vi "CSV_Image_Data_Create.vi"() -> ()   [LabVIEW 2022 SP3]
uses:
  <vilib>/Utility/file.llb/Write Delimited Spreadsheet (string).vi
panel:
  out "error out":errorcluster
  in  "error in (no error)":errorcluster
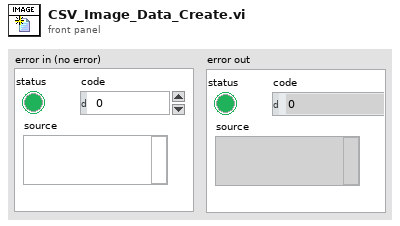
[diagram p1: front panel]
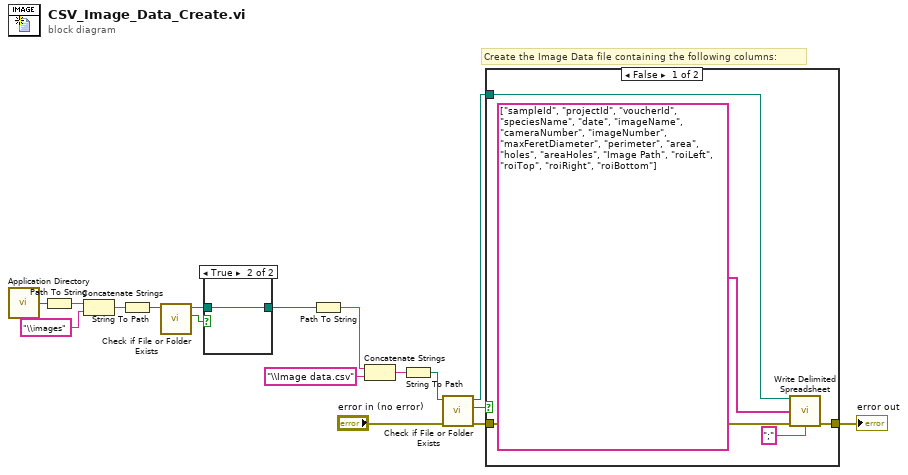
[diagram p0: block diagram]
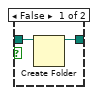
[diagram p2: hidden frame]
diagram:
  # "Create the Image Data file containing the following columns:"
  n1 = call <vilib>:"Application Directory.vi"() -> ("Application Directory"=w8:path)
  n2 = Path To String(path=w8) -> (string=w7:string)
  n3 = Concatenate Strings(w7, "\\images") -> (w5:string)
  n4 = String To Path(string=w5) -> (path=w4:path)
  n5 = call <vilib>:"Check if File or Folder Exists.vi"("path"=w4) -> ("file or folder exists?"=w3:bool, "dup path"=w2:path)  [unwired: 8 in, 1 out]
  n6 = case shown="True" w3 {
    tunnel: w2 -> [w19 w20]
    tunnel: [w18 w20] -> w1
    frame False {
      n7 = Create Folder(path (use dialog)=w19) -> (created path=w18:path)  [unwired: 2 in, 2 out]
    }
    frame True {
    }
  }
  n8 = Path To String(path=w1) -> (string=w17:string)
  n9 = Concatenate Strings(w17, "\\Image data.csv") -> (w15:string)
  n10 = String To Path(string=w15) -> (path=w14:path)
  n11 = call <vilib>:"Check if File or Folder Exists.vi"("error in (no error)"="error in (no error)", "path"=w14) -> ("error out"=w11:errorcluster, "file or folder exists?"=w13:bool, "dup path"=w12:path)  [unwired: 7 in]
  n12 = case shown="False" w13 {
    tunnel: w12 -> [w24 _]
    tunnel: w11 -> [w23 w26]
    tunnel: [w22 w26] -> w9
    frame False {
      n13 = call-poly <vilib>:"Write Delimited Spreadsheet.vi"("file path (dialog if empty)"=w24, "1D data"=string[] ["sampleId", "projectId", "voucherId", "speciesName", "date", "imageName", "cameraNumber", "imageNumber", "maxFeretDiameter", "perimeter", "area", "holes", "areaHoles", "Image Path", "roiLeft", "roiTop", "roiRight", "roiBottom"], "error in (no error)"=w23, "delimiter (\\t)"=";" ("delimiter (\\t)")) -> ("error out"=w22:errorcluster)  [unwired: 10 in, 1 out]
    }
    frame True {
    }
  }
  "error out" <- w9
